vi "Prime Pump.vi"(6 "Cycles":u16=5, 8 "error in (no error)":errorcluster, 9 "Waste Valve Pos.":u16=2, 10 "Buffer Val Pos.":u16=3, 11 "Autosampler in":refnum<class "Autosampler.lvclass">) -> (0 "error out":errorcluster, 3 "Autosampler out":refnum<class "Autosampler.lvclass">)   [LabVIEW 2023, in "Autosampler.lvlib" / "Autosampler.lvclass"]
uses:
  Autosampler.lvclass
  Autosampler.lvclass/Autosampler.ctl
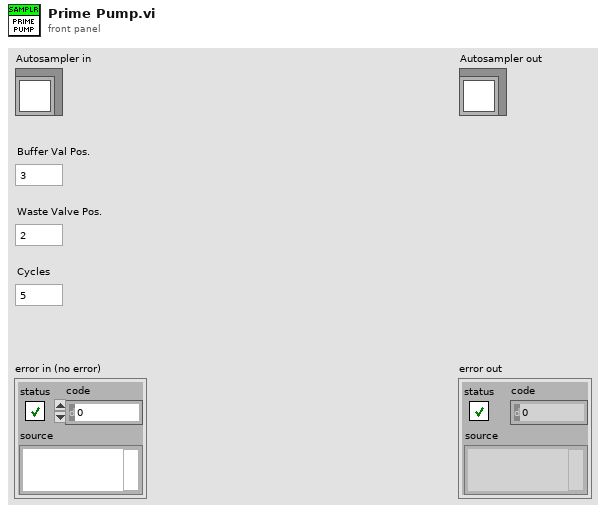
[diagram p1: front panel]
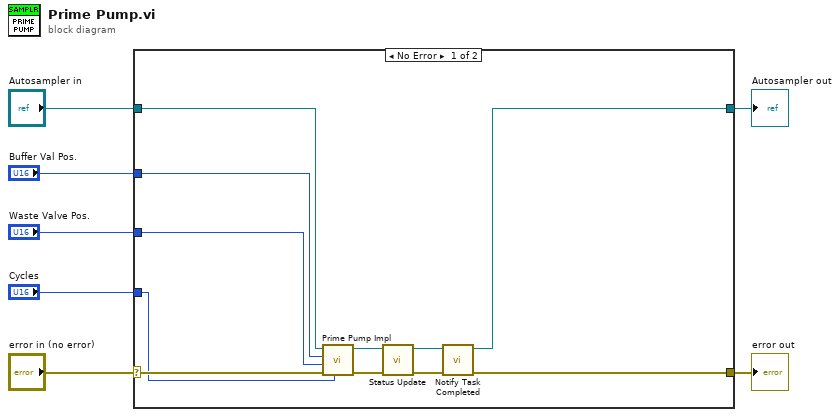
[diagram p0: block diagram]
diagram:
  n1 = case shown="No Error" "error in (no error)" {
    selector: "error in (no error)" -> [w17 w20]
    tunnel: [w15 w20] -> w6
    tunnel: [w11 w19] -> w4
    tunnel: "Autosampler in" -> [w14 w19]
    tunnel: "Cycles" -> [w8 _]
    tunnel: "Waste Valve Pos." -> [w9 _]
    tunnel: "Buffer Val Pos." -> [w10 _]
    frame No Error {
      n2 = call-dynamic "Prime Pump Impl.vi"("Cycles"=w8, "error in (no error)"=w17, "Waste Valve Pos."=w9, "Buffer Val Pos."=w10, "Autosampler in"=w14) -> ("error out"=w18:errorcluster, "Autosampler out"=w12:refnum<class "Autosampler.lvclass">)  [unwired: 5 in]
      n3 = call "Status Update.vi"("error in (no error)"=w18, "Autosampler in"=w12) -> ("error out"=w16:errorcluster, "Autosampler out"=w13:refnum<class "Autosampler.lvclass">)  [unwired: 7 in, 1 out]
      n4 = call-dynamic "Notify Task Completed.vi"("error in (no error)"=w16, "Device in"=w13) -> ("error out"=w15:errorcluster, "Device out"=w11:refnum<class "Autosampler.lvclass">)  [unwired: 8 in]
    }
    frame Error {
    }
  }
  "error out" <- w6
  "Autosampler out" <- w4
